vi "Set ErrorList Qref.vi"(8 "error in (no error)":errorcluster, 10 "ErrorList Qref":refnum<queue>, 11 "ErrorHandler in":refnum<class "ErrorHandler.lvclass">) -> (0 "error out":errorcluster, 3 "ErrorHandler out":refnum<class "ErrorHandler.lvclass">)   [LabVIEW 2019, in "ErrorHandler.lvclass"]
doc: "Developed by Kevin Thompson\nkevin@thompsonengineering.net\n\nCopyright 2018\nThompson Engineering, LLC"
uses:
  ErrorHandler.lvclass
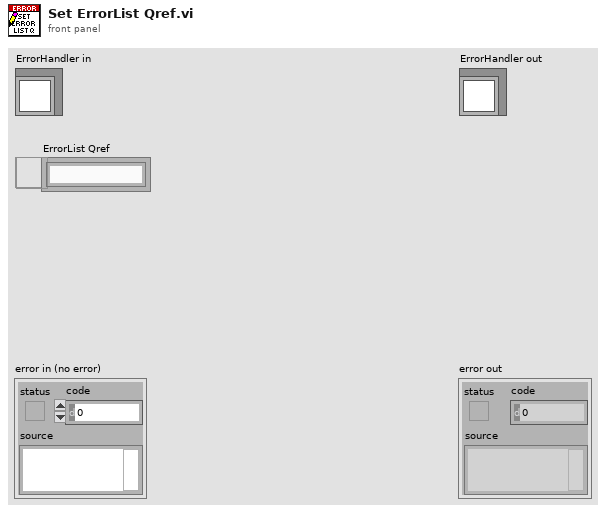
[diagram p1: front panel]
types:
  T1 = typedef "ErrorHandler.lvclass/ObjData--cluster.ctl" = cluster{"AppName":string, "ErrorLogBasePath":path, "ErrorDialogPopUp Disabled":bool, "TerminateAppOnError Enabled":bool, "Public Events":T2, "ErrorList Qref":refnum<queue>}
  T2 = typedef "ErrorHandler.lvclass/Public Events.ctl" = cluster{"ErrorRemote Ev":refnum<user-event>}
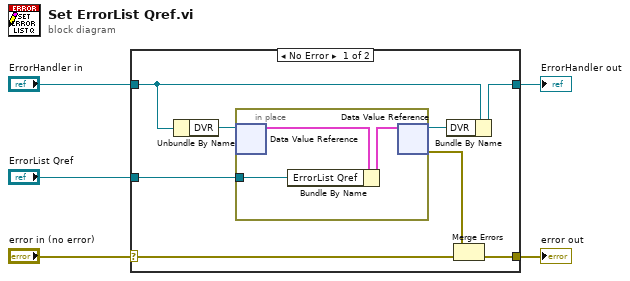
[diagram p0: block diagram]
diagram:
  n1 = case shown="No Error" "error in (no error)" {
    selector: "error in (no error)" -> [w6 w17]
    tunnel: [w8 w17] -> w4
    tunnel: [w10 w18] -> w2
    tunnel: "ErrorHandler in" -> [w9 w18]
    tunnel: "ErrorList Qref" -> [w7 _]
    frame No Error {
      n2 = Unbundle By Name(w9) -> ("DVR"=w11:refnum<data-value>)
      n3 = in-place {
        in-place-border: w7 -> [w16]
        n4 = in-place-dvr #1(w11) -> (w15:T1)  [unwired: 1 out]
        n5 = Bundle By Name(cluster=w15, "ErrorList Qref"=w16) -> (w14:T1)
        n6 = in-place-dvr #1(w14) -> (w13:refnum<data-value>, w12:errorcluster)
      }
      n7 = Bundle By Name(cluster=w9, "DVR"=w13) -> (w10:refnum<class "ErrorHandler.lvclass">)
      n8 = Merge Errors(w12, w6) -> (w8:errorcluster)
    }
    frame Error {
    }
  }
  "error out" <- w4
  "ErrorHandler out" <- w2
